vi "Prototype.vi"(8 "error in (no error)":errorcluster, 10 "User Defined Prototype in":refnum<class "User Defined Prototype.lvclass">, 11 "Scripter in":refnum<class "Message Scripter.lvclass">) -> (0 "error out":errorcluster, 2 "User Defined Prototype out":refnum<class "User Defined Prototype.lvclass">, 3 "Scripter out":refnum<class "Message Scripter.lvclass">)   [LabVIEW 2020, in "Message Maker.lvlib" / "User Defined Prototype.lvclass"]
uses:
  User Defined Prototype.lvclass
  Message Maker.lvlib
  Message Scripter/Message Scripter.lvclass
  Abstract Icon Prototyper/Abstract Icon Prototyper.lvclass
  Prototyper/Prototyper.lvclass
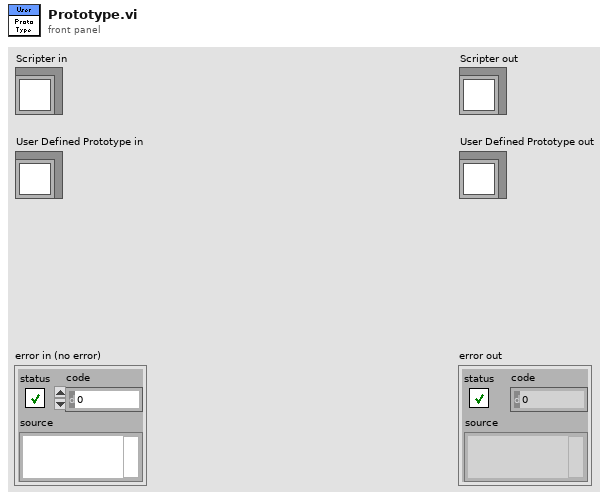
[diagram p1: front panel]
types:
  T1 = enum16{"Invalid Wire Rule", "Required", "Recommended", "Optional", "Dynamic Dispatch"}[]
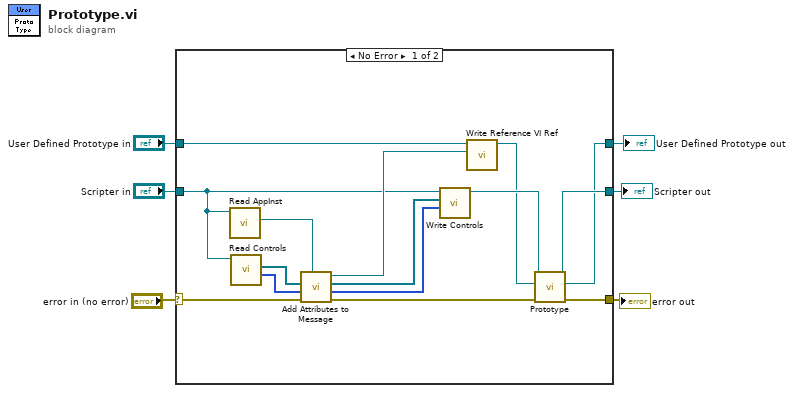
[diagram p0: block diagram]
diagram:
  n1 = case shown="No Error" "error in (no error)" {
    selector: "error in (no error)" -> [w7 w24]
    tunnel: [w17 w24] -> w6
    tunnel: [w15 w23] -> w5
    tunnel: [w14 w22] -> w4
    tunnel: "User Defined Prototype in" -> [w13 w22]
    tunnel: "Scripter in" -> [w8 w23]
    frame No Error {
      n2 = call "Read AppInst.vi"("Message Maker in"=w8) -> ("AppInst"=w21:refnum<vi>)  [unwired: 10 in]
      n3 = call "Read Controls.vi"("Message Scripter in"=w8) -> ("Wiring Rules"=w9:T1, "Controls[]"=w10:refnum<vi>[])  [unwired: 9 in]
      n4 = call "Add Attributes to Message.vi"("AppInst"=w21, "error in (no error)"=w7, "Original Wiring Rules"=w9, "Original Controls"=w10) -> ("error out"=w18:errorcluster, "Wiring Rules"=w20:T1, "Controls"=w19:refnum<vi>[], "Scratch VI Ref"=w11:refnum<vi>)  [unwired: 4 in]
      n5 = call "Write Controls.vi"("Wiring Rules"=w20, "Controls[]"=w19, "Message Scripter in"=w8) -> ("Message Scripter out"=w16:refnum<class "Message Scripter.lvclass">)  [unwired: 8 in]
      n6 = call "Write Reference VI Ref.vi"("Reference VI Ref"=w11, "Prototyper in"=w13) -> ("Prototyper out"=w12:refnum<class "User Defined Prototype.lvclass">)  [unwired: 9 in]
      n7 = call-parent "Prototype.vi"("error in (no error)"=w18, "Abstract Prototyper in"=w12, "Scripter in"=w16) -> ("error out"=w17:errorcluster, "Abstract Prototyper out"=w14:refnum<class "User Defined Prototype.lvclass">, "Scripter out"=w15:refnum<class "Message Scripter.lvclass">)  [unwired: 6 in]
    }
    frame Error {
    }
  }
  "error out" <- w6
  "User Defined Prototype out" <- w4
  "Scripter out" <- w5
